vi "Add Items to All VIs Containing Moded TypeDefs Tree.vi"(8 "error in":errorcluster, 10 "Dependent TypeDefs wParents":T1[](array[typedef]), 11 "TreeControl in":refnum<vi>) -> (0 "error out":errorcluster)   [LabVIEW 2013, in "DiscoverCommonTypeDefCallers.lvlib"]
uses:
  DiscoverCommonTypeDefCallers.lvlib
  Controls/DependendentTypeDefwParents.ctl
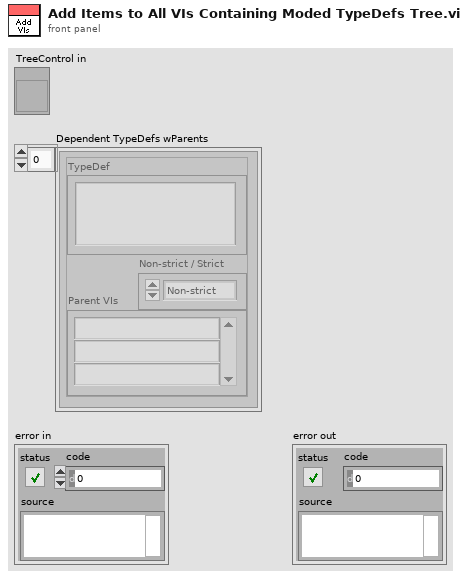
[diagram p1: front panel]
types:
  T1 = typedef "DiscoverCommonTypeDefCallers.lvlib/DependendentTypeDefwParents.ctl" = cluster{"TypeDef":string, "Non-strict / Strict":enum32{"Non-strict", "Strict"}, "Parent VIs":string[]}
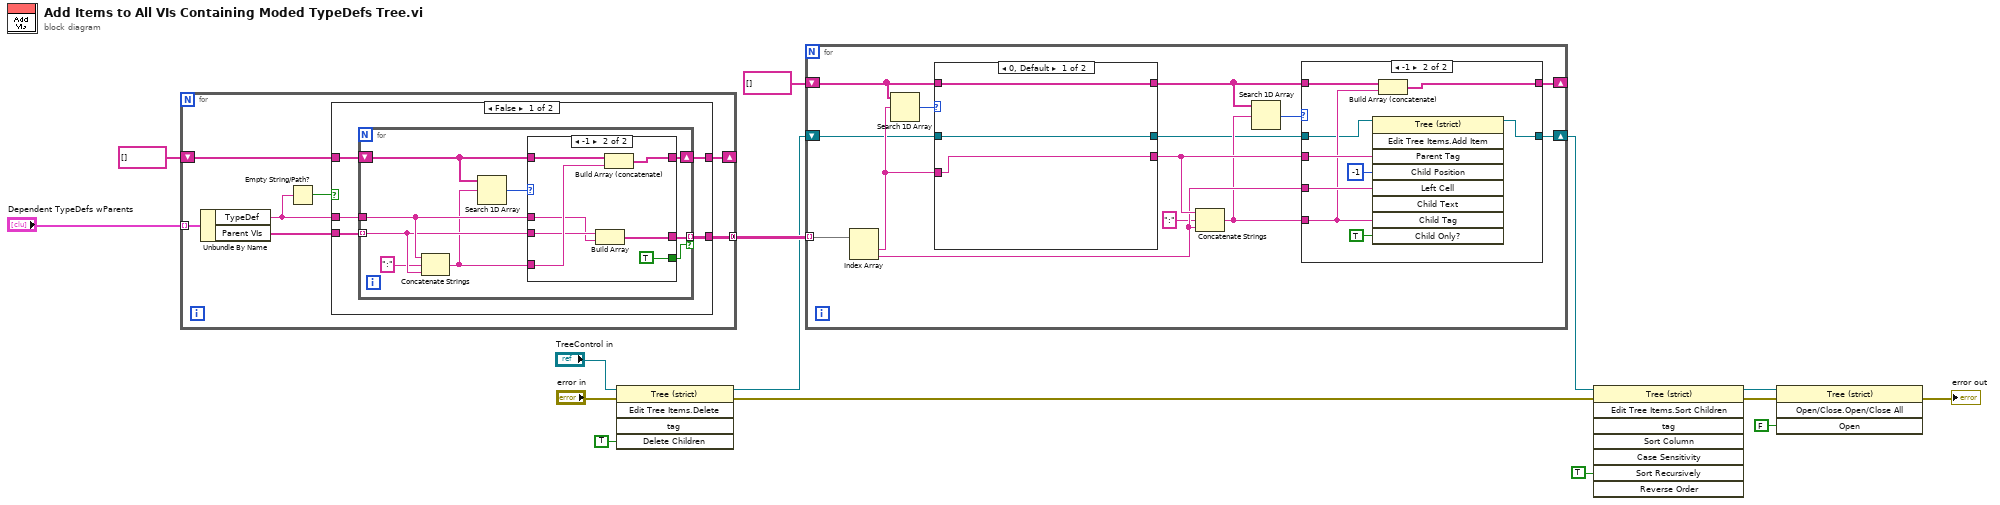
[diagram p0: block diagram]
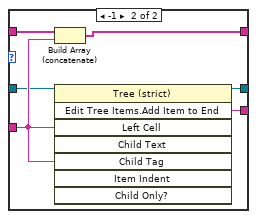
[diagram p3: hidden frame]
diagram:
  n1 = for {
    tunnel: "Dependent TypeDefs wParents" -> [w22] mode=indexing
    shift-right: [w17] -> _
    shift-left: string[] [] ("Parent VIs") -> [w18]
    tunnel: [w16] -> w12 mode=concatenating
    n2 = Unbundle By Name(w22) -> ("TypeDef"=w20:string, "Parent VIs"=w21:string[])
    n3 = Empty String/Path?(string/path=w20) -> (empty?=w19:bool)
    n4 = case shown="False" w19 {
      tunnel: w20 -> [w26 _]
      tunnel: w21 -> [w27 _]
      tunnel: w18 -> [w24 w45]
      tunnel: [w25 w45] -> w17
      tunnel: [w23 _] -> w16
      frame False {
        n5 = for {
          tunnel: w26 -> [w36]
          tunnel: w27 -> [w35] mode=indexing
          shift-right: [w32] -> w25
          shift-left: w24 -> [w33]
          tunnel: [w29] -> w23 mode=indexing if=w28
          n6 = Concatenate Strings(w36, ":" ("string"), w35) -> (w31:string)
          n7 = Search 1D Array(1D array=w33, element=w31) -> (index of element=w30:i32)  [unwired: 1 in]
          n8 = case shown="-1" w30 {
            tunnel: w36 -> [_ w40]
            tunnel: w35 -> [_ w41]
            tunnel: w33 -> [w37 w44]
            tunnel: [w37 w43] -> w32
            tunnel: w31 -> [_ w42]
            tunnel: [_ w39] -> w29
            tunnel: [_ TRUE] -> w28
            frame 0, Default {
            }
            frame -1 {
              n9 = Build Array(w41, w40) -> (w39:string[])
              n10 = Build Array (concatenate)(w44, w42) -> (w43:string[])
            }
          }
        }
      }
      frame True {
      }
    }
  }
  n11 = invoke on="Invoke Node" class="Tree (strict)" method="Edit Tree Items.Delete"(reference="TreeControl in", error in="error in", "Delete Children"=TRUE ("Delete Children?")) -> (reference out=w7:refnum<vi>, error out=w5:errorcluster)  [unwired: 2 in, 3 out]
  n12 = for {
    shift-right: [w58] -> _
    shift-left: string[] [] ("Parent VIs") -> [w59]
    tunnel: w12 -> [w54] mode=indexing
    shift-right: [w46] -> w6
    shift-left: w7 -> [w48]
    n13 = Index Array(array=w54) -> (element #1=w53:string, element #2=w52:string)  [unwired: 2 in]
    n14 = Search 1D Array(1D array=w59, element=w53) -> (index of element=w56:i32)  [unwired: 1 in]
    n15 = case shown="0, Default" w56 {
      tunnel: [w72 w79] -> w57
      tunnel: w59 -> [w73 w78]
      tunnel: w53 -> [w72 w76]
      tunnel: [w73 w77] -> w55
      tunnel: w48 -> [w71 w75]
      tunnel: [w71 w74] -> w47
      frame 0, Default {
      }
      frame -1 {
        n16 = Build Array (concatenate)(w78, w76) -> (w77:string[])
        n17 = invoke on="Invoke Node" class="Tree (strict)" method="Edit Tree Items.Add Item to End"(reference=w75, "Left Cell"=w76, "Child Tag"=w76) -> (reference out=w74:refnum<vi>, "Edit Tree Items:Add Item to End"=w79:string)  [unwired: 5 in, 6 out]
      }
    }
    n18 = Concatenate Strings(w57, ":" ("string"), w52) -> (w50:string)
    n19 = Search 1D Array(1D array=w55, element=w50) -> (index of element=w49:i32)  [unwired: 1 in]
    n20 = case shown="-1" w49 {
      tunnel: w57 -> [_ w69]
      tunnel: w52 -> [_ w68]
      tunnel: w55 -> [w61 w67]
      tunnel: [w61 w66] -> w58
      tunnel: w50 -> [_ w65]
      tunnel: w47 -> [w60 w63]
      tunnel: [w60 w62] -> w46
      frame 0, Default {
      }
      frame -1 {
        n21 = invoke on="Invoke Node" class="Tree (strict)" method="Edit Tree Items.Add Item"(reference=w63, "Parent Tag"=w69, "Child Position"=-1, "Left Cell"=w68, "Child Tag"=w65, "Child Only?"=TRUE) -> (reference out=w62:refnum<vi>)  [unwired: 3 in, 8 out]
        n22 = Build Array (concatenate)(w67, w65) -> (w66:string[])
      }
    }
  }
  n23 = invoke on="Invoke Node" class="Tree (strict)" method="Edit Tree Items.Sort Children"(reference=w6, error in=w5, "Sort Recursively"=TRUE ("Sort Recursively?")) -> (reference out=w3:refnum<vi>, error out=w2:errorcluster)  [unwired: 5 in, 6 out]
  n24 = invoke on="Invoke Node" class="Tree (strict)" method="Open/Close.Open/Close All"(reference=w3, error in=w2, "Open"=FALSE ("Open?")) -> (error out=→"error out":errorcluster)  [unwired: 1 in, 3 out]
